vi "Close.vi"(8 "error in (no error)":errorcluster, 11 "object in":refnum<class "Fetch Waveforms CFG.lvclass">) -> (0 "error out":errorcluster, 3 "object out":refnum<class "Fetch Waveforms CFG.lvclass">)   [LabVIEW 2023, in "Scope Simulated CFGs.lvlib" / "Fetch Waveforms CFG.lvclass"]
uses:
  Fetch Waveforms CFG.lvclass
  Configuration/Configuration Semaphore/CFG Semaphore.lvclass
  Fetch Waveforms CFG.lvclass/Fetch Waveforms CFG.ctl
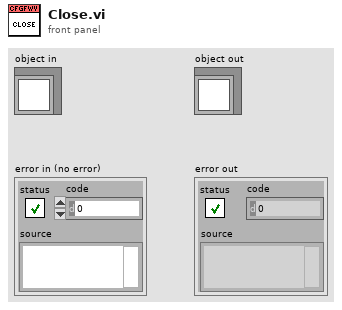
[diagram p1: front panel]
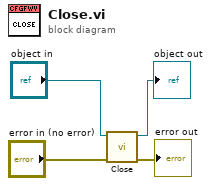
[diagram p0: block diagram]
diagram:
  n1 = call-parent "Close.vi"("error in"="error in (no error)", "CFG Semaphore in"="object in") -> ("error out"=→"error out":errorcluster, "CFG Semaphore out"=→"object out":refnum<class "Fetch Waveforms CFG.lvclass">)  [unwired: 8 in]
